vi "AlmostEqual.vi"(1 "Y":dbl, 2 "Tolerance (0.01)":dbl=0.01, 3 "X":dbl) -> (0 "X = Y":bool)   [LabVIEW 2014, in "OutputToFilePlugins.lvlib" / "OutputToFileBasePlugin.lvclass"]
uses:
  OutputToFileBasePlugin.lvclass
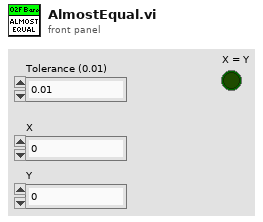
[diagram p1: front panel]
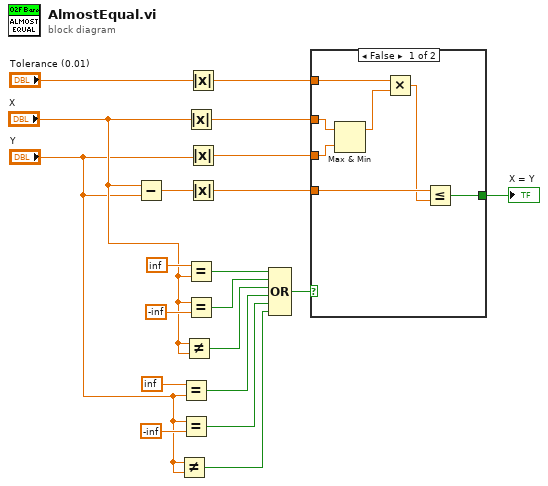
[diagram p0: block diagram]
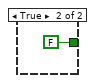
[diagram p2: hidden frame]
diagram:
  n1 = Subtract(x="X", y="Y") -> (x-y=w6:dbl)
  n2 = Not Equal?(x="Y", y="Y") -> (x != y?=w15:bool)
  n3 = Equal?(x=inf, y="Y") -> (x = y?=w13:bool)
  n4 = Equal?(x="Y", y=-inf) -> (x = y?=w14:bool)
  n5 = Not Equal?(x="X", y="X") -> (x != y?=w12:bool)
  n6 = Absolute Value(x="X") -> (abs(x)=w4:dbl)
  n7 = Equal?(x=inf, y="X") -> (x = y?=w16:bool)
  n8 = Equal?(x="X", y=-inf) -> (x = y?=w11:bool)
  n9 = Absolute Value(x="Tolerance (0.01)") -> (abs(x)=w5:dbl)
  n10 = Absolute Value(x="Y") -> (abs(x)=w3:dbl)
  n11 = Absolute Value(x=w6) -> (abs(x)=w2:dbl)
  n12 = Compound Arithmetic op=OR(w16, w11, w12, w13, w14, w15) -> (w9:bool)
  n13 = case shown="False" w9 {
    tunnel: w5 -> [w25 _]
    tunnel: w4 -> [w26 _]
    tunnel: w3 -> [w27 _]
    tunnel: w2 -> [w23 _]
    tunnel: [w21 FALSE] -> w1
    frame False {
      n14 = Max & Min(x=w26, y=w27) -> (max(x,y)=w24:dbl)  [unwired: 1 out]
      n15 = Multiply(x=w25, y=w24) -> (x*y=w22:dbl)
      n16 = Less Or Equal?(x=w23, y=w22) -> (x <= y?=w21:bool)
    }
    frame True {
    }
  }
  "X = Y" <- w1
